vi "Scale.vi"(8 "error in":errorcluster, 11 "Detail Graph in":refnum<class "Graph with Section Views.lvclass">) -> (0 "error out":errorcluster, 3 "Detail Graph out":refnum<class "Graph with Section Views.lvclass">)   [LabVIEW 2023, in "Graph with Section Views.lvclass"]
uses:
  Graph with Section Views.lvclass
  Graph with Section Views.lvclass/Graph with Section Views.ctl
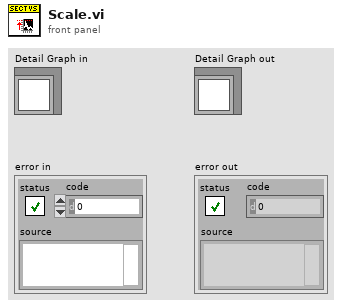
[diagram p1: front panel]
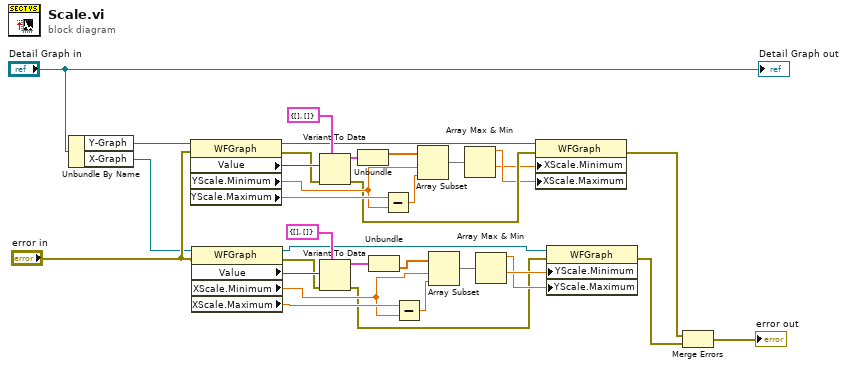
[diagram p0: block diagram]
diagram:
  n1 = Unbundle By Name("Detail Graph in") -> ("Y-Graph"=w30:refnum<vi>, "X-Graph"=w16:refnum<vi>)
  n2 = property class="WFGraph"(reference=w30, error in="error in") -> (reference out=w21:refnum<vi>, error out=w22:errorcluster, "Value"=w29:variant, "YScale.Minimum"=w24:dbl, "YScale.Maximum"=w25:dbl)
  n3 = property class="WFGraph"(reference=w16, error in="error in") -> (reference out=w9:refnum<vi>, error out=w5:errorcluster, "Value"=w14:variant, "XScale.Minimum"=w7:dbl, "XScale.Maximum"=w8:dbl)
  n4 = Variant To Data(error in=w22, type=cluster{dbl[], dbl[]} {[], []} ("cluster"), Variant=w29) -> (data=w27:cluster{dbl[], dbl[]}, error out=w20:errorcluster)
  n5 = Variant To Data(error in=w5, type=cluster{dbl[], dbl[]} {[], []} ("cluster"), Variant=w14) -> (data=w2:cluster{dbl[], dbl[]}, error out=w6:errorcluster)
  n6 = Unbundle(w27) -> (w26:dbl[])  [unwired: 1 out]
  n7 = Unbundle(w2) -> (w1:dbl[])  [unwired: 1 out]
  n8 = Subtract(x=w25, y=w24) -> (x-y=w23:dbl)
  n9 = Subtract(x=w8, y=w7) -> (x-y=w10:dbl)
  n10 = Array Subset(array=w26, index=w24, length=w23) -> (w19:dbl[])
  n11 = Array Subset(array=w1, index=w7, length=w10) -> (w11:dbl[])
  n12 = Array Max & Min(array=w19) -> (max value=w18:dbl, min value=w17:dbl)  [unwired: 2 out]
  n13 = Array Max & Min(array=w11) -> (max value=w12:dbl, min value=w13:dbl)  [unwired: 2 out]
  n14 = property class="WFGraph"(reference=w21, error in=w20, "XScale.Minimum"=w17, "XScale.Maximum"=w18) -> (error out=w3:errorcluster)  [unwired: 1 out]
  n15 = property class="WFGraph"(reference=w9, error in=w6, "YScale.Minimum"=w13, "YScale.Maximum"=w12) -> (error out=w4:errorcluster)  [unwired: 1 out]
  n16 = Merge Errors(w3, w4) -> (→"error out":errorcluster)
  "Detail Graph out" <- "Detail Graph in"
